vi "test-cubic-spline-02.vi"() -> ()   [LabVIEW 2019]
uses:
  <vilib>/Rock Robotics/WPI/ThirdParty/JAS_Junk/TrajLib/POSEwCURVATURE.ctl
  <vilib>/Rock Robotics/WPI/ThirdParty/JAS_Junk/TrajLib/POSE2D.ctl
  <vilib>/Rock Robotics/WPI/ThirdParty/JAS_Junk/TrajLib/TRANSLATION2D.ctl
  <vilib>/Rock Robotics/WPI/ThirdParty/JAS_Junk/TrajLib/ROTATION2D.ctl
  <vilib>/Rock Robotics/WPI/ThirdParty/JAS_Junk/TrajLib/Rotation_CreateAngle.vi
  <vilib>/Rock Robotics/WPI/ThirdParty/JAS_Junk/TrajLib/Util_CalcDist.vi
  <vilib>/Rock Robotics/WPI/ThirdParty/JAS_Junk/TrajLib/Trajectory_Library.lvlib
panel:
  out "XY Graph":cluster{dbl[], dbl[]}(graph)
  out "All Interior \nwayPoints\nFound (True)":bool
  out "end rot = 0":dbl
  out "end y = 0":dbl
  out "end x = 0":dbl
  out "start rot = 0":dbl
  out "start y = 0":dbl
  out "start x = 0":dbl
  out "max dtheta < 0.0872":dbl
  out "max dy < 0.00127":dbl
  out "max dx  < 0.127":dbl
  out "Overall Error":errorcluster
  out "Elements":i32
  out "Create Spline Error":errorcluster
  out "SplinePoses\nWCurve":T1[](array[typedef]) {"POSE"."ROTATION"."SIN" format="%13.4f"; "POSE"."ROTATION"."COS" format="%13.4f"; "POSE"."ROTATION"."VALUE" format="%13.4f"; "POSE"."TRANSLATION"."Y" format="%14.3f"; "POSE"."TRANSLATION"."X" format="%14.3f"}
  out "Elapsed Time":dbl
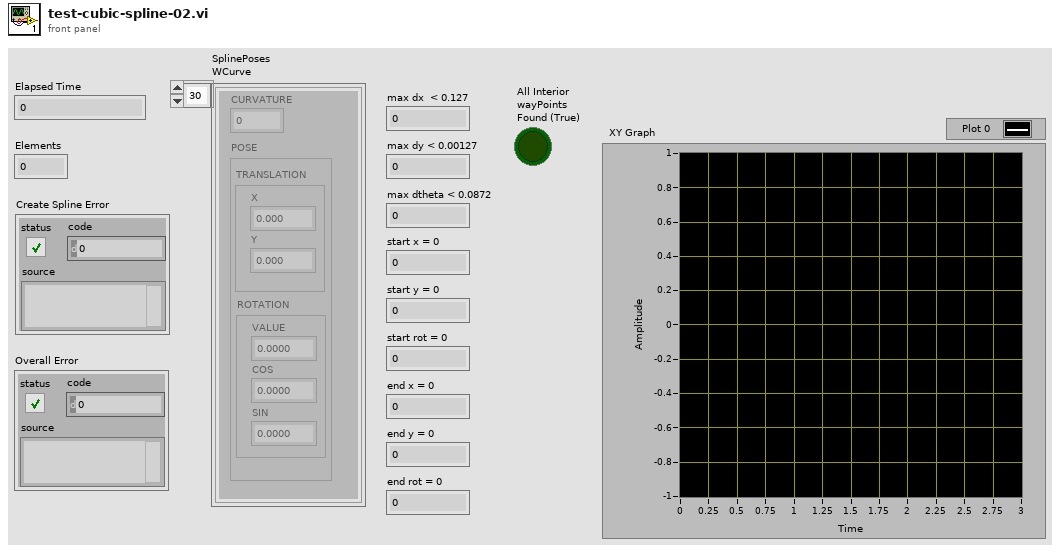
[diagram p1: front panel]
types:
  T1 = typedef "Trajectory_Library.lvlib/POSEwCURVATURE.ctl" = cluster{"CURVATURE":dbl, "POSE":T2}
  T2 = typedef "Trajectory_Library.lvlib/POSE2D.ctl" = cluster{"TRANSLATION":T3, "ROTATION":T4}
  T3 = typedef "Trajectory_Library.lvlib/TRANSLATION2D.ctl" = cluster{"X":dbl, "Y":dbl}
  T4 = typedef "Trajectory_Library.lvlib/ROTATION2D.ctl" = cluster{"VALUE":dbl, "COS":dbl, "SIN":dbl}
  T5 = typedef "Trajectory_Library.lvlib/SPLINE_CTRL_VECTOR.ctl" = cluster{"Xs":dbl[], "Ys":dbl[]}
  T6 = typedef "Trajectory_Library.lvlib/SPLINE.ctl" = cluster{"Degree":i32, "Coefficients":T7}
  T7 = typedef "NI_Matrix.lvlib/RealMatrix.ctl" = dbl[][]
  T8 = typedef "Trajectory_Library.lvlib/TWIST2D.ctl" = cluster{"dX":dbl, "dY":dbl, "dTHETA":dbl}
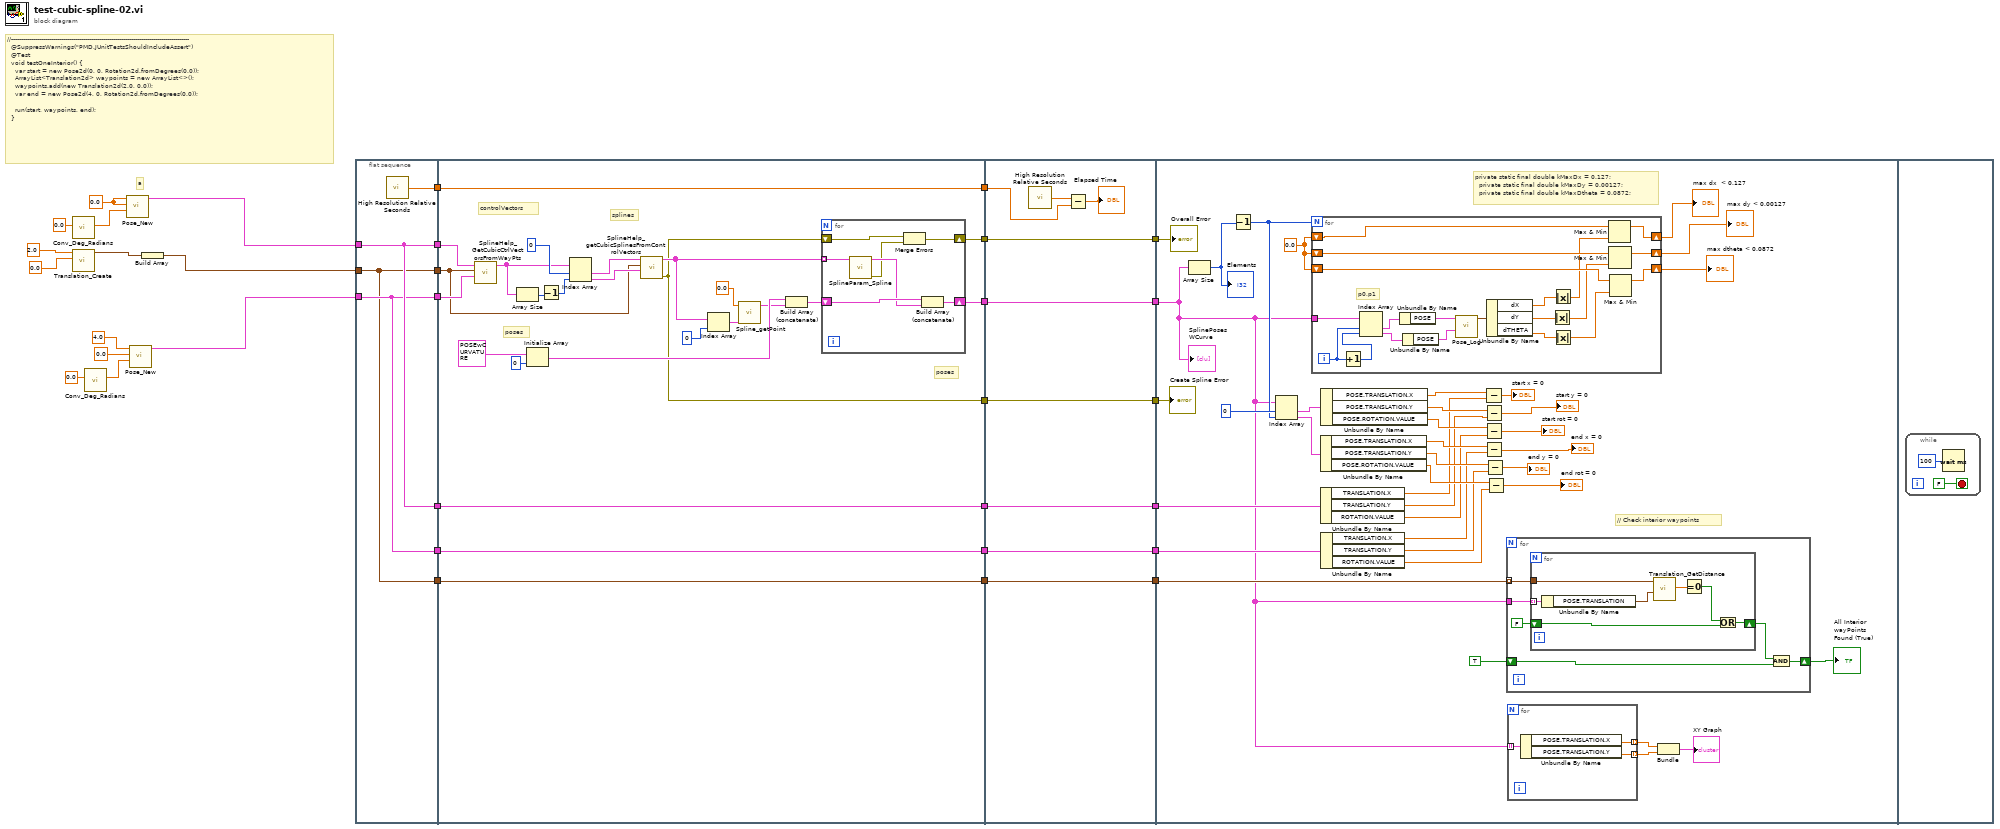
[diagram p0: block diagram]
diagram:
  w9 = 0.0 ("X")
  # "a"
  # "//-----------------------------------------------------------------------------------------\n  @SuppressWarnings(\"PMD.JUnitTestsShouldIncludeAssert\")\n  @Test\n  void testOneInterior() {\n    var start = new Pose2d(0, 0, Rotation2d.fromDegrees(0.0));\n    ArrayList<Translation2d> waypoints = new ArrayList<>();\n    waypoints.add(new Translation2d(2.0, 0.0));\n    var end = new Pose2d(4, 0, Rotation2d.fromDegrees(0.0));\n\n    run(start, waypoints, end);\n  }"
  n1 = call <vilib>:"Conv_Deg_Radians.vi"("Degress"=0.0) -> ("Radians"=w8:dbl)  [unwired: 10 in]
  n2 = call <vilib>:"Translation_Create.vi"("Y"=0.0, "X"=2.0) -> ("TRANSLATION"=w5:T3)  [unwired: 9 in]
  n3 = call <vilib>:"Conv_Deg_Radians.vi"("Degress"=0.0) -> ("Radians"=w1:dbl)  [unwired: 10 in]
  n4 = call <vilib>:"Pose_New.vi"("Heading"=w8, "Y"=w9, "X"=w9) -> ("out POSe"=w31:T2)  [unwired: 8 in]
  n5 = call <vilib>:"Pose_New.vi"("Heading"=w1, "Y"=0.0, "X"=4.0) -> ("out POSe"=w28:T2)  [unwired: 8 in]
  n6 = Build Array(w5) -> (w6:T3[])
  n7 = flat-sequence {
    tunnel: w31 -> [w36]
    tunnel: [w36] -> w30
    tunnel: w6 -> [w34]
    tunnel: [w34] -> w29
    tunnel: w28 -> [w35]
    tunnel: [w35] -> w27
    tunnel: [w37] -> w26
    tunnel: [w36] -> w18
    tunnel: [w35] -> w15
    tunnel: [w34] -> w10
    tunnel: w30 -> [w62]
    tunnel: w29 -> [w54]
    tunnel: w27 -> [w61]
    tunnel: [w53] -> w25
    tunnel: w26 -> [w53]
    tunnel: [w43] -> w24
    tunnel: [w42] -> w22
    tunnel: [w41] -> w20
    tunnel: w18 -> [w40]
    tunnel: [w40] -> w17
    tunnel: w15 -> [w39]
    tunnel: [w39] -> w14
    tunnel: [w38] -> w11
    tunnel: w10 -> [w38]
    tunnel: w25 -> [w78]
    tunnel: w24 -> [w77]
    tunnel: [w77] -> w23
    tunnel: w22 -> [w76]
    tunnel: [w76] -> w21
    tunnel: w20 -> [w75]
    tunnel: [w75] -> w19
    tunnel: w17 -> [w72]
    tunnel: [w72] -> w16
    tunnel: w14 -> [w71]
    tunnel: [w71] -> w13
    tunnel: [w70] -> w12
    tunnel: w11 -> [w70]
    tunnel: w23 -> [w79]
    tunnel: w21 -> [w116]
    tunnel: w19 -> [w115]
    tunnel: w16 -> [w109]
    tunnel: w13 -> [w108]
    tunnel: w12 -> [w85]
    frame #0 {
      n8 = call <vilib>:"High Resolution Relative Seconds.vi"() -> ("relative seconds"=w37:dbl)
    }
    frame #1 {
      # "poses"
      # "poses"
      # "splines"
      # "controlVectors"
      n9 = call <vilib>:"SplineHelp_GetCubicCtrlVectorsFromWayPts.vi"("Enging POSE"=w61, "Interior WAYPOINTS"=w54, "Starting POSE"=w62) -> ("SplineControlVectors"=w58:T5[])  [unwired: 8 in]
      n10 = Array Size(array=w58) -> (size(s)=w59:i32)
      n11 = Initialize Array(T1 {"CURVATURE"=0.0, "POSE"={"TRANSLATION"={"X"=0.0, "Y"=0.0}, "ROTATION"={"VALUE"=0.0, "COS"=1.0, "SIN"=0.0}}} ("POSEwCURVATURE"), 0 ("dimension size")) -> (w47:T1[])
      n12 = Decrement(x=w59) -> (x-1=w57:i32)
      n13 = Index Array(array=w58, index #1=0 ("index"), index #2=w57) -> (element #1=w56:T5, element #2=w55:T5)
      n14 = call <vilib>:"SplineHelp_getCubicSplinesFromControlVectors.vi"("endCtrlVector"=w55, "InternalWaypoints"=w54, "startCtrlVector"=w56) -> ("error out"=w42:errorcluster, "splines"=w44:T6[])  [unwired: 3 in, 4 out]
      n15 = Index Array(array=w44, index=0) -> (element=w49:T6)
      n16 = call <vilib>:"Spline_getPoint.vi"("inputSPLINE"=w49, "Time"=0.0) -> ("POSEwCURVATURE"=w46:T1)  [unwired: 9 in]
      n17 = Build Array (concatenate)(w47, w46) -> (w45:T1[])
      n18 = for {
        shift-right: [w66] -> w43
        shift-left: w45 -> [w68]
        tunnel: w44 -> [w69] mode=indexing
        shift-right: [w64] -> w41
        shift-left: w42 -> [w65]
        n19 = call <vilib>:"SplineParam_Spline.vi"("inputSPLINE"=w69) -> ("error out"=w63:errorcluster, "outputPOSEwCURVATURE"=w67:T1[])  [unwired: 9 in]
        n20 = Merge Errors(w65, w63) -> (w64:errorcluster)
        n21 = Build Array (concatenate)(w68, w67) -> (w66:T1[])
      }
    }
    frame #2 {
      n22 = call <vilib>:"High Resolution Relative Seconds.vi"() -> ("relative seconds"=w73:dbl)
      n23 = Subtract(x=w73, y=w78) -> (x-y=→"Elapsed Time":dbl)
    }
    frame #3 {
      w113 = 0.0
      # "// Check interior waypoints"
      # "private static final double kMaxDx = 0.127;\n  private static final double kMaxDy = 0.00127;\n  private static final double kMaxDtheta = 0.0872;"
      n24 = Array Size(array=w79) -> (size(s)=w114:i32)
      "Elements" <- w114
      n25 = Decrement(x=w114) -> (x-1=w106:i32)
      n26 = Index Array(array=w79, index #1=0 ("index"), index #2=w106) -> (element #1=w105:T1, element #2=w104:T1)
      n27 = for {
        N: w106 -> [_]
        tunnel: w79 -> [w150]
        shift-right: [w141] -> w112
        shift-left: w113 -> [w138]
        shift-right: [w139] -> w110
        shift-left: w113 -> [w136]
        shift-right: [w140] -> w111
        shift-left: w113 -> [w137]
        i -> [w152]
        # "p0,p1"
        n28 = Increment(x=w152) -> (x+1=w151:i32)
        n29 = Index Array(array=w150, index #1=w152, index #2=w151) -> (element #1=w149:T1, element #2=w148:T1)
        n30 = Unbundle By Name(w149) -> ("POSE"=w147:T2)
        n31 = Unbundle By Name(w148) -> ("POSE"=w146:T2)
        n32 = call <vilib>:"Pose_Log.vi"("end POSE"=w146, "in POSE"=w147) -> ("out TWIST"=w145:T8)  [unwired: 9 in]
        n33 = Unbundle By Name(w145) -> ("dX"=w142:dbl, "dY"=w143:dbl, "dTHETA"=w144:dbl)
        n34 = Absolute Value(x=w143) -> (abs(x)=w134:dbl)
        n35 = Absolute Value(x=w142) -> (abs(x)=w135:dbl)
        n36 = Absolute Value(x=w144) -> (abs(x)=w133:dbl)
        n37 = Max & Min(x=w138, y=w135) -> (max(x,y)=w141:dbl)  [unwired: 1 out]
        n38 = Max & Min(x=w137, y=w134) -> (max(x,y)=w140:dbl)  [unwired: 1 out]
        n39 = Max & Min(x=w136, y=w133) -> (max(x,y)=w139:dbl)  [unwired: 1 out]
      }
      "max dx  < 0.127" <- w112
      "max dy < 0.00127" <- w111
      "max dtheta < 0.0872" <- w110
      n40 = Unbundle By Name(w104) -> ("POSE.TRANSLATION.X"=w100:dbl, "POSE.TRANSLATION.Y"=w99:dbl, "POSE.ROTATION.VALUE"=w98:dbl)
      n41 = Unbundle By Name(w109) -> ("TRANSLATION.X"=w97:dbl, "TRANSLATION.Y"=w96:dbl, "ROTATION.VALUE"=w95:dbl)
      n42 = Unbundle By Name(w105) -> ("POSE.TRANSLATION.X"=w103:dbl, "POSE.TRANSLATION.Y"=w102:dbl, "POSE.ROTATION.VALUE"=w101:dbl)
      n43 = Unbundle By Name(w108) -> ("TRANSLATION.X"=w94:dbl, "TRANSLATION.Y"=w93:dbl, "ROTATION.VALUE"=w92:dbl)
      n44 = Subtract(x=w103, y=w97) -> (x-y=→"start x = 0":dbl)
      n45 = Subtract(x=w102, y=w96) -> (x-y=→"start y = 0":dbl)
      n46 = Subtract(x=w101, y=w95) -> (x-y=→"start rot = 0":dbl)
      n47 = Subtract(x=w100, y=w94) -> (x-y=→"end x = 0":dbl)
      n48 = Subtract(x=w99, y=w93) -> (x-y=→"end y = 0":dbl)
      n49 = Subtract(x=w98, y=w92) -> (x-y=→"end rot = 0":dbl)
      n50 = for {
        tunnel: w85 -> [w120] mode=indexing
        tunnel: w79 -> [w125]
        shift-right: [w124] -> w83
        shift-left: TRUE -> [w123]
        n51 = for {
          tunnel: w125 -> [w129] mode=indexing
          shift-right: [w132] -> w121
          shift-left: FALSE -> [w131]
          tunnel: w120 -> [w130]
          n52 = Unbundle By Name(w129) -> ("POSE.TRANSLATION"=w128:T3)
          n53 = call <vilib>:"Translation_GetDistance.vi"("other Translation"=w128, "In Translation"=w130) -> ("Distance"=w127:dbl)  [unwired: 9 in]
          n54 = Equal To 0?(x=w127) -> (x = 0?=w126:bool)
          n55 = Or(x=w126, y=w131) -> (x .or. y?=w132:bool)
        }
        n56 = And(x=w121, y=w123) -> (x .and. y?=w124:bool)
      }
      "All Interior \nwayPoints\nFound (True)" <- w83
      n57 = for {
        tunnel: [w119] -> w82 mode=indexing
        tunnel: [w118] -> w81 mode=indexing
        tunnel: w79 -> [w117] mode=indexing
        n58 = Unbundle By Name(w117) -> ("POSE.TRANSLATION.X"=w119:dbl, "POSE.TRANSLATION.Y"=w118:dbl)
      }
      n59 = Bundle(w82, w81) -> (→"XY Graph":cluster{dbl[], dbl[]})  [unwired: 1 in]
      "SplinePoses\nWCurve" <- w79
      "Create Spline Error" <- w116
      "Overall Error" <- w115
    }
    frame #4 {
      n60 = while {
        stop <- FALSE stop-if-true
        n61 = Wait (ms)(milliseconds to wait=u32 100) -> ()  [unwired: 1 out]
      }
    }
  }
